vi "VisaBasicForSolder.vi"(1 "VISA resource name":refnum<visa-resource-name>, 2 "Cmd":string, 3 "TimeOut":bool=TRUE, 4 "Time(0.1)":u32=10, 5 "error in (no error)":errorcluster, 8 "VisaAction":enum16{"Open", "Send", "Recieve", "Close"}(ring)) -> (16 "read string":string, 19 "error out":errorcluster)   [LabVIEW 2019]
uses:
  <vilib>/Instr/_visa.llb/VISA Configure Serial Port (Instr).vi
  LLB/Commonly VI.lvlib
panel:
  # "? --> 827D B2"
  # "FE62 B1"
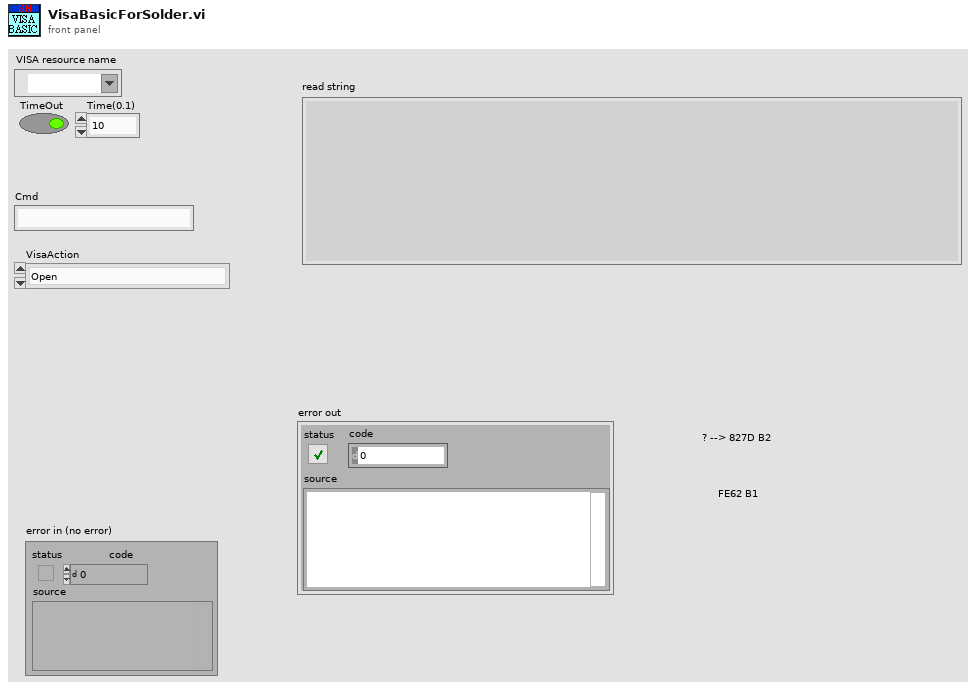
[diagram p1: front panel]
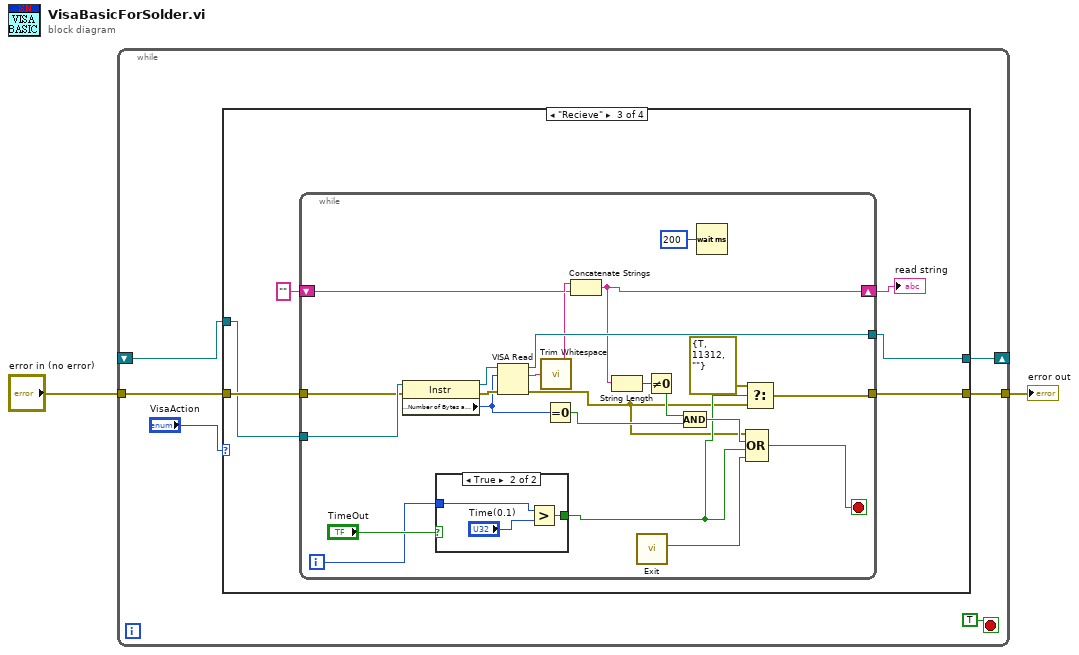
[diagram p0: block diagram]
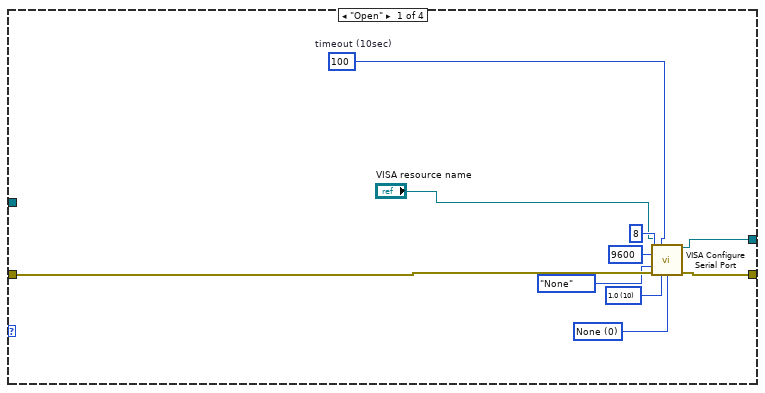
[diagram p2: hidden frame]
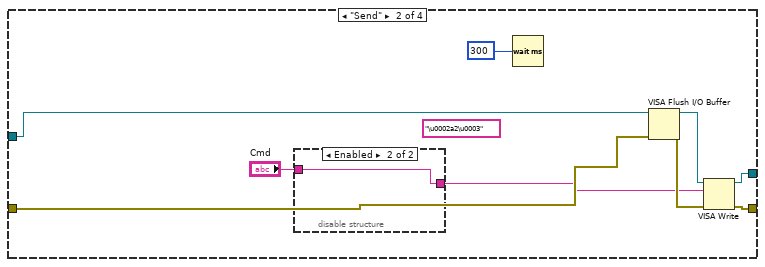
[diagram p3: hidden frame]
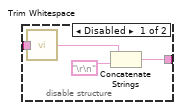
[diagram p4: hidden frame]
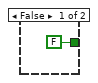
[diagram p5: hidden frame]
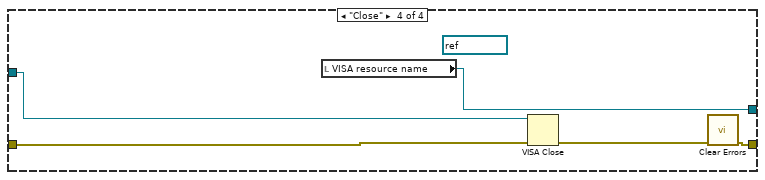
[diagram p6: hidden frame]
diagram:
  n1 = while {
    tunnel: "error in (no error)" -> [w6]
    tunnel: [w7] -> w2
    shift-right: [w4] -> _
    shift-left: _ -> [w3]
    stop <- TRUE stop-if-true
    n2 = case shown="\"Recieve\"" "VisaAction" {
      tunnel: [w18 w27 w37 w67] -> w7
      tunnel: w6 -> [w17 w21 w38 w69]
      tunnel: w3 -> [_ w22 w33 w68]
      tunnel: [w10 w25 w35 w66] -> w4
      frame "Open" {
        w12 = u16 0 items=["None", "XON/XOFF", "RTS/CTS", "XON/XOFF & RTS/CTS", "DTR/DSR", "XON/XOFF & DTR/DSR"] ("flow control (0:none)")
        w13 = u16 10 items=["1.0"=10, "1.5"=15, "2.0"=20] ("stop bits (10: 1 bit)")
        w16 = u32 100  # timeout (10sec)
        n3 = call-poly "VISA Configure Serial Port"("VISA resource name"="VISA resource name", "timeout (10sec)"=w16, "baud rate (9600)"=u32 9600, "data bits (8)"=u16 8, "parity (0:none)"=enum16{"None", "Odd", "Even", "Mark", "Space"}."None", "error in (no error)"=w17, "stop bits (10: 1 bit)"=w13, "flow control (0:none)"=w12) -> ("VISA resource name out"=w10:refnum<visa-resource-name>, "error out"=w18:errorcluster)  [unwired: 1 in, 5 out]
      }
      frame "Send" {
        (unwired) "\u0002a2\u0003"
        n4 = disable-structure shown="Enabled" {
          disable-tunnel: "Cmd" -> [w31 w32]
          disable-tunnel: [w30 w32] -> w19
          frame Disabled {
            n5 = call <vilib>:"Trim Whitespace.vi"("string"=w31) -> ("trimmed string"=w28:string)  [unwired: 1 in]
            n6 = Concatenate Strings(w28, "\r\n") -> (w30:string)
          }
          frame Enabled {
          }
        }
        n7 = Wait (ms)(milliseconds to wait=u32 300 ("millisecond timer value")) -> ()  [unwired: 1 out]
        n8 = VISA Flush I/O Buffer(VISA resource name=w22, error in (no error)=w21) -> (VISA resource name out=w23:refnum<visa-resource-name>, error out=w24:errorcluster)  [unwired: 1 in]
        n9 = VISA Write(VISA resource name=w23, write buffer=w19, error in (no error)=w24) -> (VISA resource name out=w25:refnum<visa-resource-name>, error out=w27:errorcluster)  [unwired: 1 out]
      }
      frame "Recieve" {
        n10 = while {
          tunnel: w33 -> [w59]
          tunnel: w38 -> [w58]
          tunnel: [w57] -> w35
          tunnel: [w53] -> w37
          shift-right: [w39] -> w34
          shift-left: "" ("trimmed string") -> [w56]
          i -> [w43]
          stop <- w54 stop-if-true
          n11 = property class="Instr"(reference=w59, error in=w58) -> (reference out=w60:refnum<visa-resource-name>, error out=w61:errorcluster, "Serial Settings:Number of Bytes at Serial Port"=w44:u32)
          n12 = case shown="True" "TimeOut" {
            tunnel: w43 -> [_ w65]
            tunnel: [FALSE w63] -> w42
            frame False {
            }
            frame True {
              n13 = Greater?(x=w65, y="Time(0.1)") -> (0:w63:bool)
            }
          }
          n14 = VISA Read(VISA resource name=w60, byte count=w44, error in (no error)=w61) -> (VISA resource name out=w57:refnum<visa-resource-name>, read buffer=w46:string, error out=w41:errorcluster)  [unwired: 1 out]
          n15 = call <vilib>:"Trim Whitespace.vi"("string"=w46) -> ("trimmed string"=w40:string)  [unwired: 1 in]
          n16 = Equal To 0?(x=w44) -> (x = 0?=w51:bool)
          n17 = Concatenate Strings(w56, w40) -> (w39:string)
          n18 = String Length(string=w39) -> (length=w50:i32)
          n19 = call "Exit.vi"() -> ("ExitOut"=w47:bool)  [unwired: 11 in]
          n20 = Not Equal To 0?(x=w50) -> (x != 0?=w49:bool)
          n21 = Compound Arithmetic op=AND(w49, w51) -> (w48:bool)
          n22 = Wait (ms)(milliseconds to wait=u32 200) -> ()  [unwired: 1 out]
          n23 = Select(t=errorcluster {"status"=TRUE, "code"=11312, "source"=""}, s=w42, f=w41) -> (s? t:f=w53:errorcluster)
          n24 = Compound Arithmetic op=OR(w41, w48, w42, w47) -> (w54:bool)
        }
        "read string" <- w34
      }
      frame "Close" {
        (unwired) refnum<visa-resource-name> "COM3" ("VISA resource name out")
        n25 = local read "VISA resource name"() -> (w66:refnum<visa-resource-name>)
        n26 = VISA Close(VISA resource name=w68, error in (no error)=w69) -> (error out=w70:errorcluster)
        n27 = call <vilib>:"Clear Errors.vi"("error in (no error)"=w70) -> ("error out"=w67:errorcluster)  [unwired: 5 in, 1 out]
      }
    }
  }
  "error out" <- w2
